vi "DoPaint.vi"(8 "error in (no error)":errorcluster, 11 "Black in":refnum<class "Black.lvclass">) -> (0 "error out":errorcluster, 3 "Black out":refnum<class "Black.lvclass">)   [LabVIEW 2014, in "Black.lvclass"]
uses:
  Black.lvclass
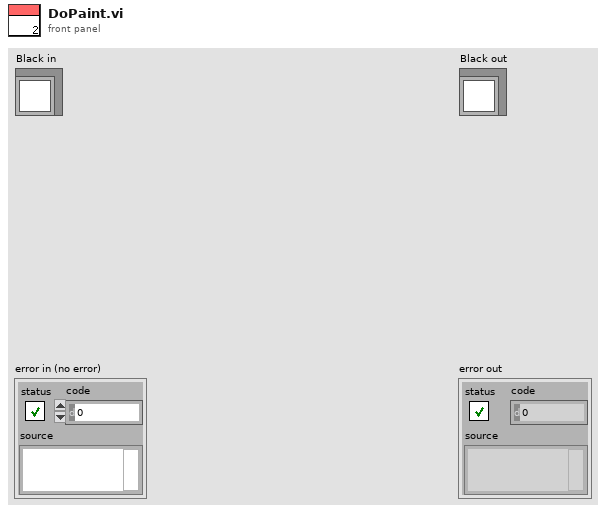
[diagram p1: front panel]
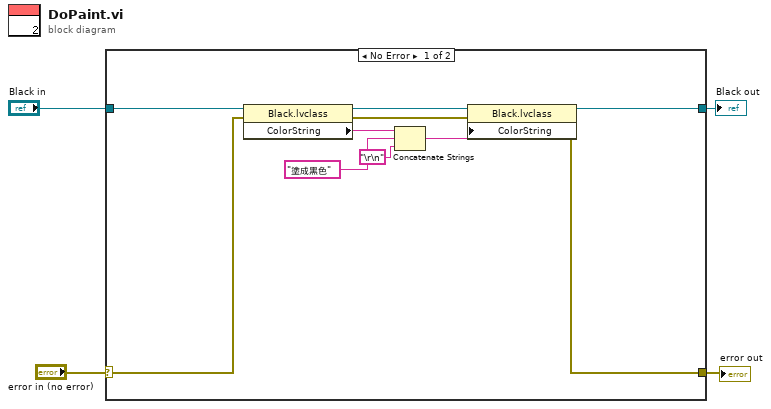
[diagram p0: block diagram]
diagram:
  n1 = case shown="No Error" "error in (no error)" {
    selector: "error in (no error)" -> [w14 w16]
    tunnel: [w11 w16] -> w4
    tunnel: [w9 w15] -> w3
    tunnel: "Black in" -> [w12 w15]
    frame No Error {
      n2 = property class="Black.lvclass"(reference=w12, error in=w14) -> (reference out=w10:refnum<class "Black.lvclass">, error out=w13:errorcluster, "ColorString"=w8:string)
      n3 = Concatenate Strings(w8, "塗成黑色" ("string"), "\r\n" ("string")) -> (w7:string)
      n4 = property class="Black.lvclass"(reference=w10, error in=w13, "ColorString"=w7) -> (reference out=w9:refnum<class "Black.lvclass">, error out=w11:errorcluster)
    }
    frame Error {
    }
  }
  "error out" <- w4
  "Black out" <- w3
